vi "NotARefNum.vi"(3 "reference in":refnum<class "G#Interface.lvclass">) -> (0 "not a refnum?":bool, 1 "reference out":refnum<class "G#Interface.lvclass">)   [LabVIEW 2020, in "G#Interface.lvclass"]
doc: "Checks if the specified object reference is valid."
uses:
  G#Interface.lvclass
  G#Interface.lvclass/G#Interface.ctl
  G#Object/G#Object.lvclass
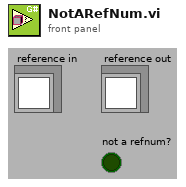
[diagram p1: front panel]
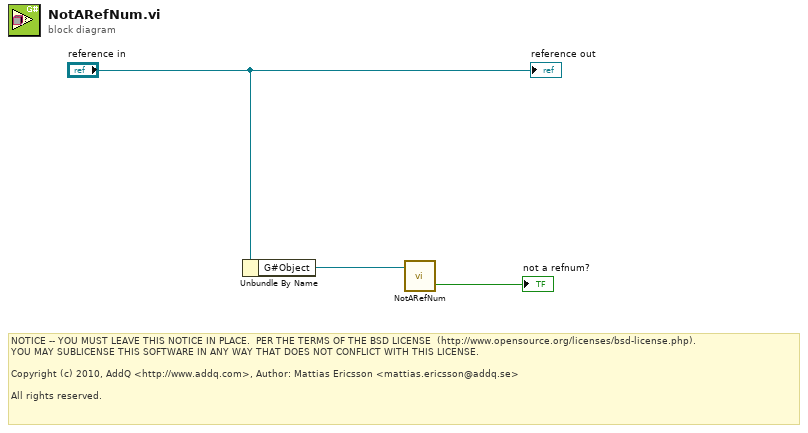
[diagram p0: block diagram]
diagram:
  # "NOTICE -- YOU MUST LEAVE THIS NOTICE IN PLACE.  PER THE TERMS OF THE BSD LICENSE  (http://www.opensource.org/licenses/bsd-license.php).\nYOU MAY SUBLICENSE THIS SOFTWARE IN ANY WAY THAT DOES NOT CONFLICT WITH THIS LICENSE.\n\nCopyright (c) 2010, AddQ <http://www.addq.com>, Author: Mattias Ericsson <mattias.ericsson@addq.se>\n\nAll rights reserved."
  n1 = Unbundle By Name("reference in") -> ("G#Object"=w2:refnum<class "G#Object.lvclass">)
  n2 = call-dynamic "NotARefNum.vi"("reference in"=w2) -> ("not a refnum?"=→"not a refnum?":bool)  [unwired: 1 in, 1 out]
  "reference out" <- "reference in"
